vi "Calc - WBmeas.vi"(9 "A":dbl, 10 "C":dbl, 11 "B":dbl) -> (3 "WBMeas":dbl)   [LabVIEW 2018, in "Controller (Host).lvlib"]
uses:
  Controller (Host).lvlib
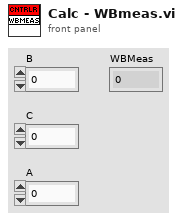
[diagram p1: front panel]
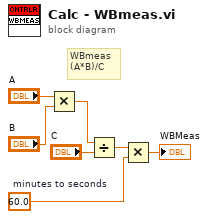
[diagram p0: block diagram]
diagram:
  w3 = 60.0  # minutes to seconds
  # "WBmeas \n(A*B)/C"
  n1 = Multiply(x="A", y="B") -> (x*y=w1:dbl)
  n2 = Divide(x=w1, y="C") -> (x/y=w2:dbl)
  n3 = Multiply(x=w2, y=w3) -> (x*y=→"WBMeas":dbl)
